vi "ConfigureTiming.vi"(0 "object in":refnum<class "AD2_MSO_SDK.lvclass">, 5 "error in (no error)":errorcluster) -> (14 "object out":refnum<class "AD2_MSO_SDK.lvclass">, 19 "error out":errorcluster)   [LabVIEW 2021, in "AD2_MSO_SDK.lvclass"]
uses:
  AD2_MSO_SDK.lvclass
  AD2_MSO_SDK.lvclass/AD2_MSO_SDK.ctl
  Olasdwf/Olasdwf.lvlib
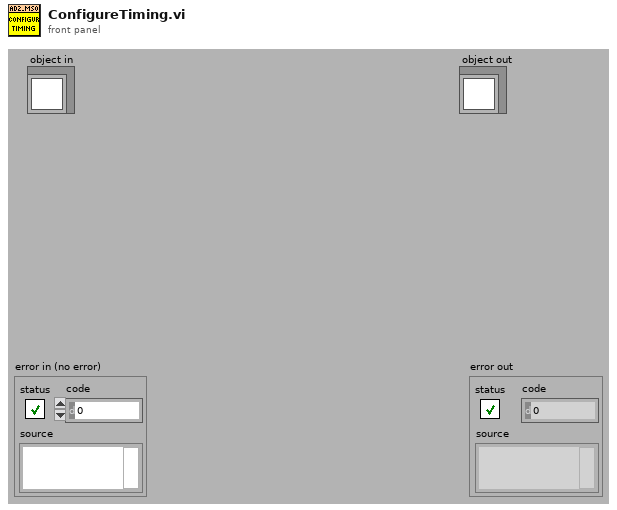
[diagram p1: front panel]
types:
  T1 = enum16{"Single Sample", "Scanshift", "Multiple Samples", "Scan Screen"}
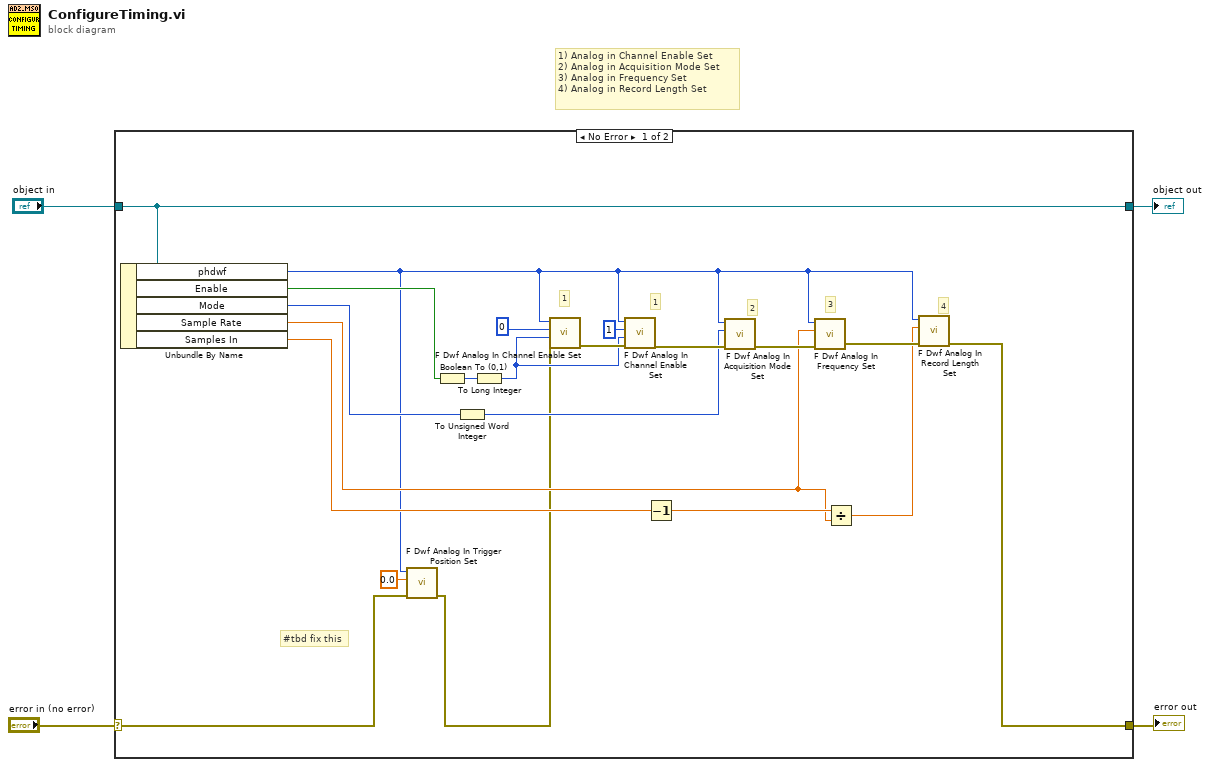
[diagram p0: block diagram]
diagram:
  # "1) Analog in Channel Enable Set\n2) Analog in Acquisition Mode Set\n3) Analog in Frequency Set\n4) Analog in Record Length Set"
  n1 = case shown="No Error" "error in (no error)" {
    selector: "error in (no error)" -> [w7 w27]
    tunnel: [w14 w27] -> w3
    tunnel: [w25 w26] -> w1
    tunnel: "object in" -> [w25 w26]
    frame No Error {
      # "#tbd fix this"
      # "4"
      # "3"
      # "2"
      # "1"
      # "1"
      n2 = Unbundle By Name(w25) -> ("phdwf"=w8:i32, "Enable"=w13:bool, "Mode"=w12:T1, "Sample Rate"=w10:dbl, "Samples In"=w9:dbl)
      n3 = call "F Dwf Analog In Trigger Position Set.vi"("error in (no error)"=w7, "secPosition"=0.0, "hdwf"=w8) -> ("error out"=w6:errorcluster)  [unwired: 7 in, 1 out]
      n4 = Boolean To (0,1)(Boolean=w13) -> (0, 1=w22:i16)
      n5 = To Unsigned Word Integer(number=w12) -> (unsigned 16bit integer=w11:u16)
      n6 = To Long Integer(number=w22) -> (32bit integer=w20:i32)
      n7 = call "F Dwf Analog In Channel Enable Set.vi"("error in (no error)"=w6, "fEnable"=w20, "idxChannel"=0, "hdwf"=w8) -> ("error out"=w21:errorcluster)  [unwired: 6 in, 1 out]
      n8 = call "F Dwf Analog In Channel Enable Set.vi"("error in (no error)"=w21, "fEnable"=w20, "idxChannel"=1, "hdwf"=w8) -> ("error out"=w19:errorcluster)  [unwired: 6 in, 1 out]
      n9 = Decrement(x=w9) -> (x-1=w16:dbl)
      n10 = call "F Dwf Analog In Acquisition Mode Set.vi"("error in (no error)"=w19, "acqmode"=w11, "hdwf"=w8) -> ("error out"=w18:errorcluster)  [unwired: 7 in, 1 out]
      n11 = call "F Dwf Analog In Frequency Set.vi"("error in (no error)"=w18, "hzFrequency"=w10, "hdwf"=w8) -> ("error out"=w17:errorcluster)  [unwired: 7 in, 1 out]
      n12 = Divide(x=w16, y=w10) -> (x/y=w15:dbl)
      n13 = call "F Dwf Analog In Record Length Set.vi"("error in (no error)"=w17, "sLength"=w15, "hdwf"=w8) -> ("error out"=w14:errorcluster)  [unwired: 7 in, 1 out]
    }
    frame Error {
    }
  }
  "error out" <- w3
  "object out" <- w1
